vi "FF_AnkleTraj.vi"(6 "Init":bool, 8 "error in (no error)":errorcluster, 9 "AnkleVelocity":dbl[](array[numeric]), 10 "AnkleInGCS":dbl[](array[numeric]), 11 "Force Field Controller in":refnum<class "ForceField.lvclass">) -> (0 "error out":errorcluster, 1 "ClosePt":dbl[](array[numeric]), 2 "Force":dbl[](array[numeric]), 3 "Force Field Controller out":refnum<class "ForceField.lvclass">, 4 "ActiveTraj":dbl[][](array[numeric]), 5 "ForceComp":dbl[](array[numeric]))   [LabVIEW 2015, in "ForceField.lvclass"]
uses:
  ForceField.lvclass
  ForceField.lvclass/ForceField.ctl
panel:
  in  "HalfWindow":i32=120
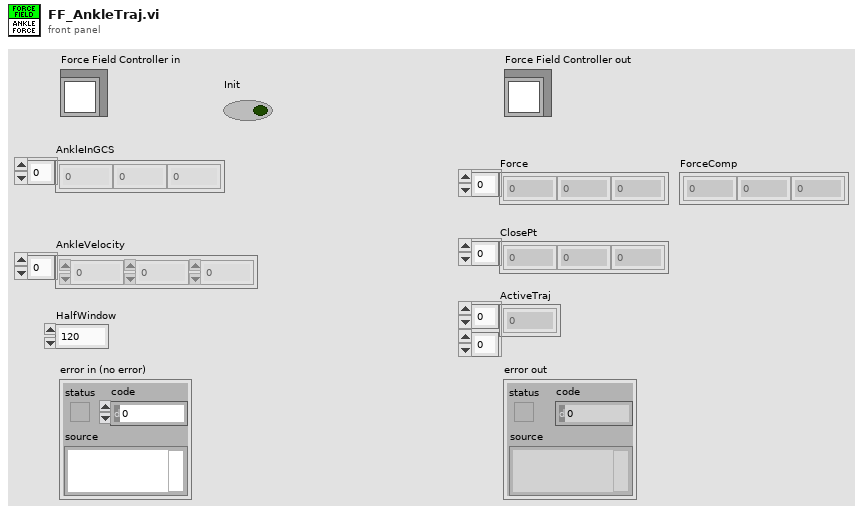
[diagram p1: front panel]
types:
  T1 = typedef "ForceField.lvclass/AnkleTrajPt.ctl" = cluster{"P1":dbl[], "P2":dbl[], "P1-P2":dbl[], "(P1-P2)^2":dbl}
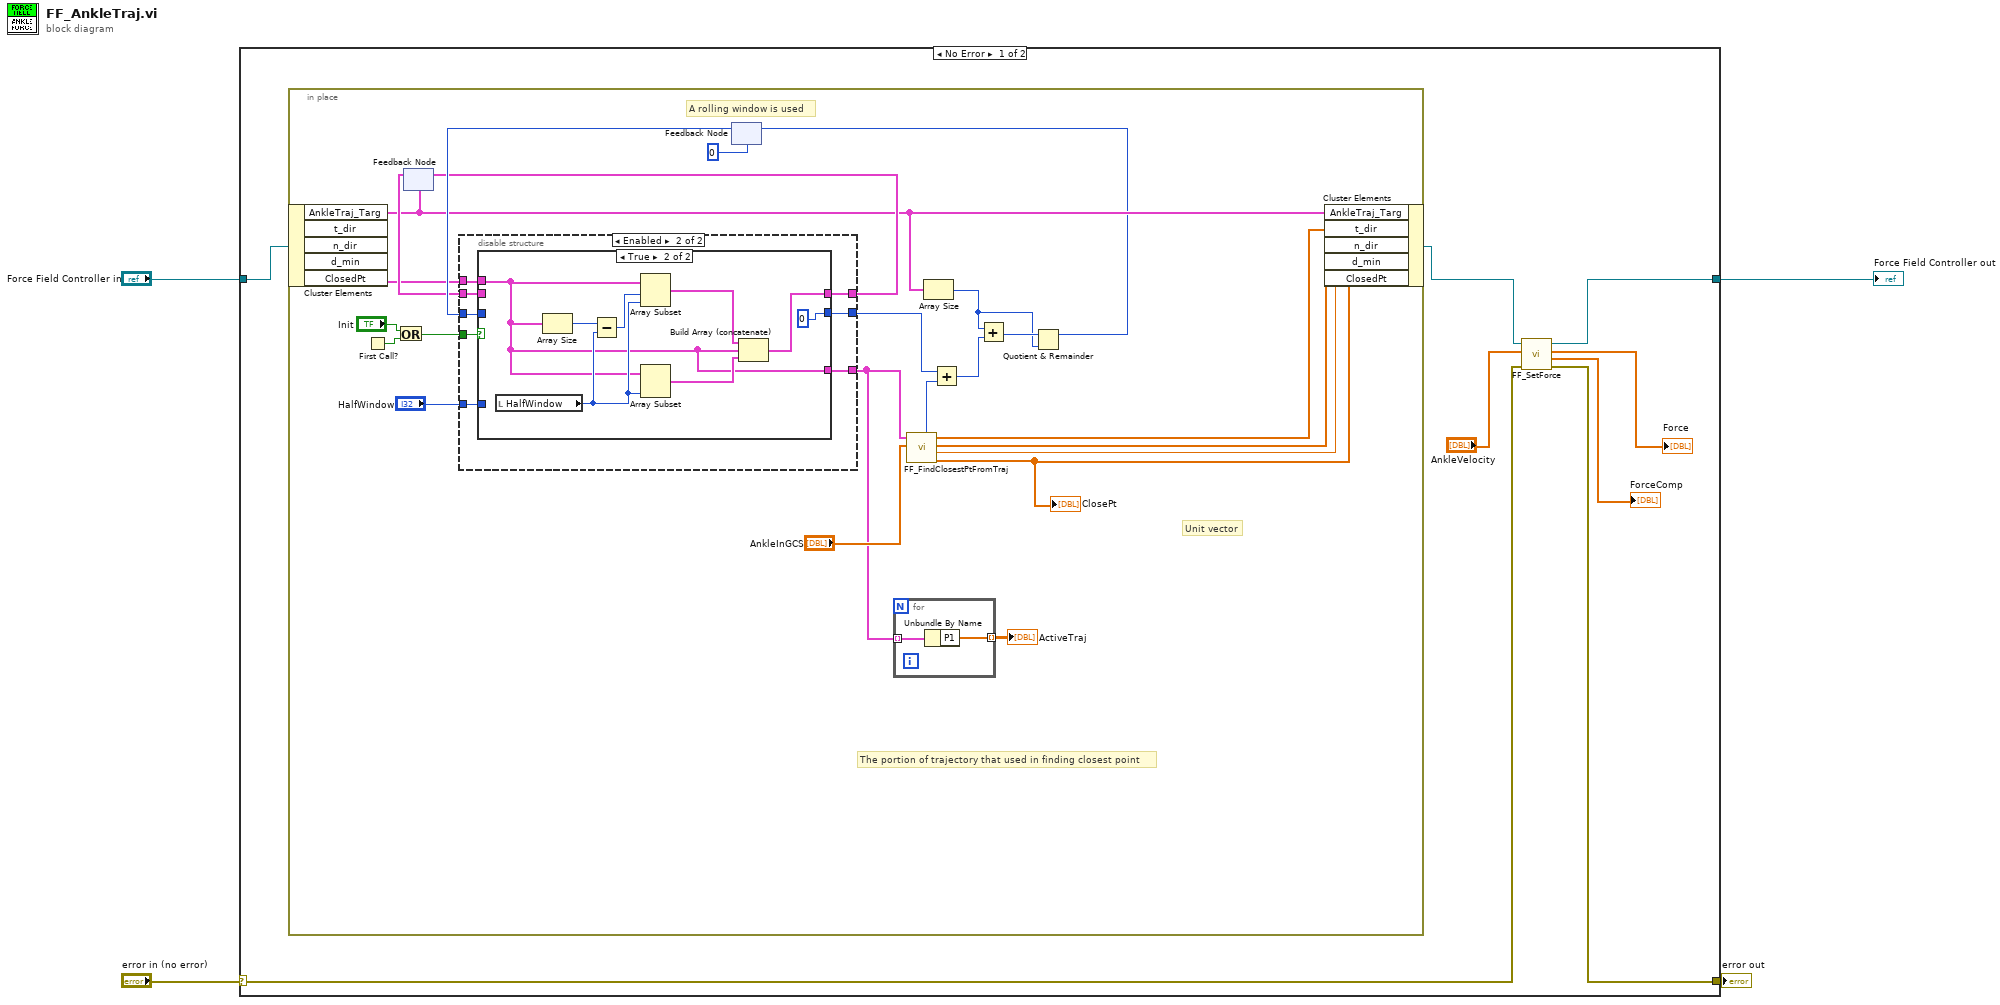
[diagram p0: block diagram]
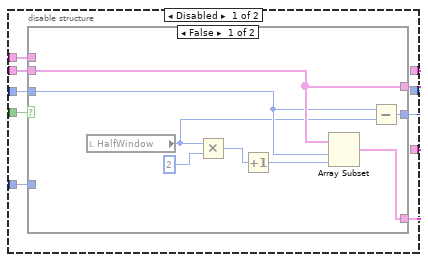
[diagram p2: hidden frame]
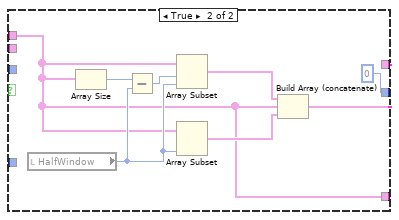
[diagram p3: hidden frame]
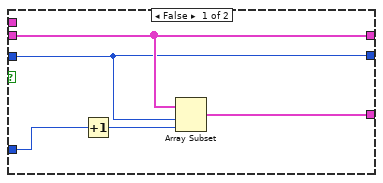
[diagram p4: hidden frame]
diagram:
  n1 = case shown="No Error" "error in (no error)" {
    selector: "error in (no error)" -> [w8 w83]
    tunnel: [w7 w83] -> w3
    tunnel: [w10 w82] -> w1
    tunnel: "Force Field Controller in" -> [w12 w82]
    frame No Error {
      n2 = in-place {
        # "A rolling window is used"
        # "The portion of trajectory that used in finding closest point"
        # "Unit vector"
        n3 = in-place-cluster #1(w12) -> ("AnkleTraj_Targ"=w27:T1[])  [unwired: 4 out]
        n4 = First Call?() -> (First Call?: T/F=w25:bool)
        n5 = Or(x="Init", y=w25) -> (x .or. y?=w23:bool)
        n6 = feedback #2(w27) -> (w30:T1[])
        n7 = feedback #3(0) -> (w32:i32)
        n8 = disable-structure shown="Enabled" {
          disable-tunnel: w23 -> [w44 w68]
          disable-tunnel: w32 -> [w43 w67]
          disable-tunnel: [w42 w66] -> w18
          disable-tunnel: w30 -> [w41 w65]
          disable-tunnel: [w40 w64] -> w29
          disable-tunnel: [w39 w63] -> w28
          disable-tunnel: w27 -> [w38 w62]
          disable-tunnel: "HalfWindow" -> [w37 w61]
          frame Disabled {
            n9 = case shown="False" w44 {
              tunnel: w43 -> [w47 _]
              tunnel: w41 -> [w51 _]
              tunnel: [w52 w53] -> w42
              tunnel: [w51 w55] -> w40
              tunnel: [w46 0] -> w39
              tunnel: w38 -> [_ w53]
              tunnel: w37 -> [_ _]
              frame False {
                n10 = local read "HalfWindow"() -> (w45:i32)
                n11 = Multiply(x=w45, y=2) -> (x*y=w50:i32)
                n12 = Increment(x=w50) -> (x+1=w49:i32)
                n13 = Array Subset(array=w51, index=w47, length=w49) -> (w52:T1[])
                n14 = Subtract(x=w47, y=w45) -> (x-y=w46:i32)
              }
              frame True {
                n15 = local read "HalfWindow"() -> (w59:i32)
                n16 = Array Size(array=w53) -> (size(s)=w60:i32)
                n17 = Subtract(x=w60, y=w59) -> (x-y=w58:i32)
                n18 = Array Subset(array=w53, index=w58, length=w59) -> (w56:T1[])
                n19 = Array Subset(array=w53, length=w59) -> (w57:T1[])  [unwired: 1 in]
                n20 = Build Array (concatenate)(w56, w53, w57) -> (w55:T1[])
              }
            }
          }
          frame Enabled {
            n21 = case shown="True" w68 {
              tunnel: w67 -> [w69 _]
              tunnel: w65 -> [w72 _]
              tunnel: [w73 w74] -> w66
              tunnel: [w72 w76] -> w64
              tunnel: [w69 0] -> w63
              tunnel: w62 -> [_ w74]
              tunnel: w61 -> [w70 _]
              frame False {
                n22 = Increment(x=w70) -> (x+1=w71:i32)
                n23 = Array Subset(array=w72, index=w69, length=w71) -> (w73:T1[])
              }
              frame True {
                n24 = local read "HalfWindow"() -> (w80:i32)
                n25 = Array Size(array=w74) -> (size(s)=w81:i32)
                n26 = Subtract(x=w81, y=w80) -> (x-y=w79:i32)
                n27 = Array Subset(array=w74, index=w79, length=w80) -> (w77:T1[])
                n28 = Array Subset(array=w74, length=w80) -> (w78:T1[])  [unwired: 1 in]
                n29 = Build Array (concatenate)(w77, w74, w78) -> (w76:T1[])
              }
            }
          }
        }
        n30 = feedback-in #2(w29) -> ()
        n31 = for {
          tunnel: w18 -> [w36] mode=indexing
          tunnel: [w35] -> w17 mode=indexing
          n32 = Unbundle By Name(w36) -> ("P1"=w35:dbl[])
        }
        "ActiveTraj" <- w17
        n33 = call "FF_FindClosestPtFromTraj.vi"("AnkleInGCS"="AnkleInGCS", "AnkleTraj"=w18) -> ("ClosestPt"=w22:dbl[], "DistanceToClosestPt"=w33:dbl, "NormalVectorToClosestPt"=w19:dbl[], "TangentVectorAtClosestPt"=w20:dbl[], "IndexOfClosePt"=w21:i32)  [unwired: 5 in]
        "ClosePt" <- w22
        n34 = Array Size(array=w27) -> (size(s)=w14:i32)
        n35 = Add(x=w28, y=w21) -> (x+y=w16:i32)
        n36 = Add(x=w14, y=w16) -> (x+y=w15:i32)
        n37 = Quotient & Remainder(x=w15, y=w14) -> (x-y*floor(x/y)=w13:i32)  [unwired: 1 out]
        n38 = feedback-in #3(w13) -> ()
        n39 = in-place-cluster #1("AnkleTraj_Targ"=w27, "t_dir"=w20, "n_dir"=w19, "d_min"=w33, "ClosedPt"=w22) -> (w11:refnum<class "ForceField.lvclass">)
      }
      n40 = call "FF_SetForce.vi"("error in (no error)"=w8, "AnkleVelocity"="AnkleVelocity", "Force Field Controller in"=w11) -> ("error out"=w7:errorcluster, "ForceNTD"=→"ForceComp":dbl[], "ForceXYZ"=→"Force":dbl[], "Force Field Controller out"=w10:refnum<class "ForceField.lvclass">)  [unwired: 5 in]
    }
    frame Error {
    }
  }
  "error out" <- w3
  "Force Field Controller out" <- w1
